vi "AgNA_Channel Trigger Sweep.vi"(8 "error in (no error)":errorcluster {"code" format="%.0x"}, 9 "TimeoutVal":i32 format="%.0g", 10 "RepCapIdentifier":string, 11 "instrument handle":refnum<k15>) -> (0 "error out":errorcluster {"code" format="%.0x"}, 3 "instrument handle out":refnum<k15>)   [LabVIEW 2015]
uses:
  <instrlib>/Agilent NA/Agilent NA.lvlib
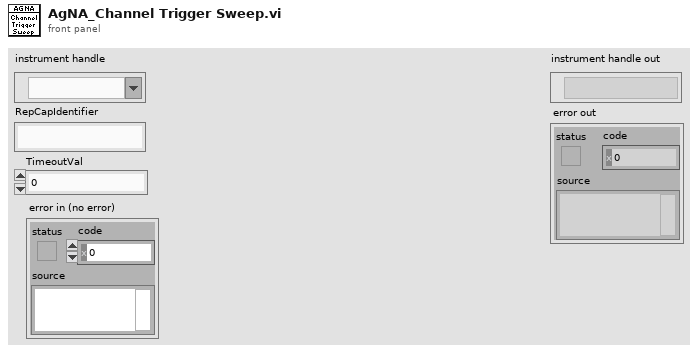
[diagram p1: front panel]
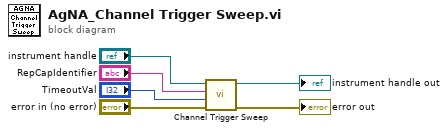
[diagram p0: block diagram]
diagram:
  n1 = call <instrlib>:"Channel Trigger Sweep.vi"("error in (no error)"="error in (no error)", "TimeoutVal"="TimeoutVal", "RepCapIdentifier"="RepCapIdentifier", "instrument handle"="instrument handle") -> ("error out"=→"error out":errorcluster, "instrument handle out"=→"instrument handle out":refnum<k15>)  [unwired: 6 in]
